vi "Save SCH FPGA Config Parameters to File MGI RWA.vi"(8 "error in (no error)":errorcluster, 11 "Refnum in":T2) -> (0 "error out":errorcluster, 2 "FPGA Configuration Values":T1={"Ln2 Filter Size"=10, "VT Quench Tick Limit"=4000000, "VT Quench Volt Limit"=0.1000061035156, "Joint Tick Limit"=4000000, "Joint Volt Limit"=0.0002000033855438, "CoWound Volt Limit"=0.2000122070312, "CoWound Tick Limit"=4000000, "SC Bus Limit"=0.0004000067710876, "SC Bus Tick Limit"=4000000, "ResMag Tick Limit"=1000000, "DAQ Cycle Ticks"=4096, "Res Mag dI/dt Delay"=256, "dI/dT scaling"=38.14697265625, "Pressure Inlet Limit (BarA)"=6.0, "Bore Tube Volt Limit"=0.5999999940395, "Pressure Outlet Limit (BarA)"=5.0, "Activation Current (kA)"=0.5, "Dump Resistor Scale Factor"=204.7939999998, "Co-Wound Asymmetry Factor"=-0.0026654, "Co-Wound Scale Factor"=60.04379999638, "Layer Scale Factors"=[4.000479996204, 3.501155003905, 3.50127799809, 3.501155003905, 3.001561000943, 3.001561000943, 3.50005300343, 3.500664994121, 3.501155003905, 4.000159993768, 3.999679997563, 4.000159993768, 3.998879998922, 3.999520003796, 3.999679997563, 4.000320002437, 4.00096000731, 4.000640004873], "Fudge Factors"=[0.0486624, 0.0491151, -0.0418637, -0.0149169, 0.0726134, -0.0451977, -0.0032112, -0.0234927, -0.002501, 0.0285479, -0.0270486, 0.003522, 0.0059306, -0.0088003, -0.0297659, 0.0390219], "Joint Scale Factors"=[0.0002005249261856, 0.0002005249261856, 0.0002004057168961, 0.000200480222702, 0.0002004057168961, 0.0002007633447647, 0.0002006888389587, 0.0002006441354752], "SC Bus Scale"=[0.09999999403954, 0.09999999403954, 0.001000002026558, 0.001000002026558, 0.0002005249261856, 0.0002006441354752], "Pressure Scale Factor"=[1.723690003157, 1.723690003157, 1.723690003157, 1.723690003157], "# Consecutive Zeros Fault"=1000, "Digitize Convert Ticks"=200, "Digitize Reset Ticks"=400, "Convert Clock Ticks"=20, "Digitize Read Delay Ticks"=38, "Digitize # Bits"=16, "HTS Lead Tick Limit"=4000000, "Res Lead Tick Limit"=4000000, "HTS Lead Trip"=0.1500000059605, "Res Lead Limit"=0.001953125, "HTS Lead FRZ"=0.006999999284744, "HTS Lead Warn"=0.001000002026558, "Low Current (kA)"=0.04500000178814, "Low Current Ticks"=400000000, "Low Current Delay Factor"=100, "HTS Resistance (nOhm)"=[0.0, 0.0], "Ticks to Close Relief"=80000000, "All Breaker Tick Limit"=400000000, "HTS Offset (microV)"=[0.0, 0.0], "Delay Ticks Between Bkr Reset"=1200000000, "Breaker Reset Ticks"=400000000, "PS Enable Reset Ticks"=400000000, "Reset Digitizer Ticks"=400000000, "Pressure Inlet Cooldown Limit"=12.0, "Pressure Outlet Cooldown Limit"=10.0, "Notification Email"="sth@magnet.fsu.edu"} {"Pressure Outlet Cooldown Limit" format="%.5g"; "Pressure Inlet Cooldown Limit" format="%.5g"; "HTS Offset (microV)" format="%_6g"; "HTS Resistance (nOhm)" format="%_6g"; "HTS Lead Warn" format="%_6g"; "HTS Lead FRZ" format="%_6g"; "Res Lead Limit" format="%_6g"; "HTS Lead Trip" format="%_6g"; "Pressure Scale Factor" format="%_6g"; "Joint Scale Factors" format="%_6g"; "Fudge Factors" format="%.7g"; "Co-Wound Asymmetry Factor" format="%.8g"; "Activation Current (kA)" format="%_6g"; "Pressure Outlet Limit (BarA)" format="%.5g"; "Bore Tube Volt Limit" format="%_6g"; "Pressure Inlet Limit (BarA)" format="%.5g"; "dI/dT scaling" format="%.11g"; "SC Bus Limit" format="%_6g"; "Joint Volt Limit" format="%_6g"; "VT Quench Volt Limit" format="%.5g"}, 3 "Refnum out":T2)   [LabVIEW 2021]
doc: "Author: Scott Hannahs <sth@magnet.fsu.edu>\nCopyright 2018 Florida State University, All rights reserved."
uses:
  RT Controls/FPGA SCH Digitizer Ref.ctl
  SCH Data Controls/FPGA Configure Parameters.ctl
  <userlib>/_MGI/Read Write Anything/MGI RWA Options Cluster.ctl
  <vilib>/Utility/error.llb/Error Cluster From Error Code.vi
  <vilib>/rvi/errors/niLvFpgaAdjustHostInterfaceError.vi
  RT Server Sub VIs/RT Host Globals.vi
  <vilib>/rvi/interface/nirviReadWriteControl/nirviReadWriteControl.xnode
  NiFpgaLv.dll
  <vilib>/rvi/interface/Simulation/niFpgaSimulationCallBeginRW.vi
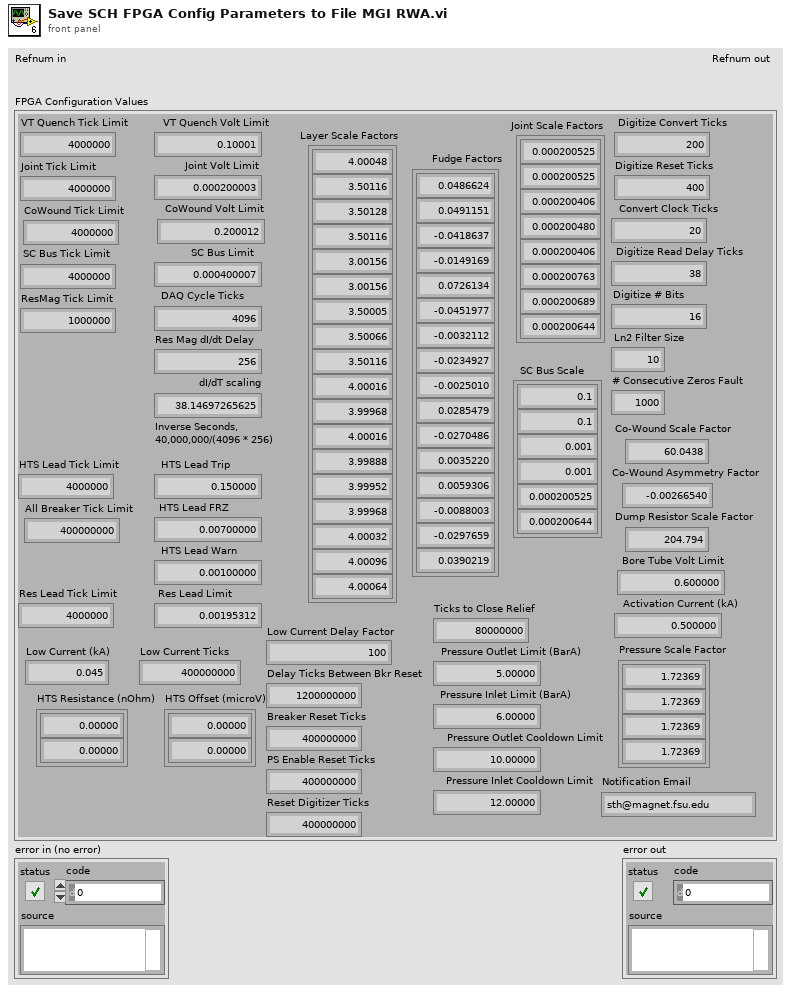
[diagram p1: front panel]
types:
  T1 = typedef "FPGA Configure Parameters.ctl" = cluster{"Ln2 Filter Size":i16, "VT Quench Tick Limit":u32, "VT Quench Volt Limit":dbl, "Joint Tick Limit":u32, "Joint Volt Limit":dbl, "CoWound Volt Limit":dbl, "CoWound Tick Limit":u32, "SC Bus Limit":dbl, "SC Bus Tick Limit":u32, "ResMag Tick Limit":u32, "DAQ Cycle Ticks":u32, "Res Mag dI/dt Delay":u32, "dI/dT scaling":dbl, "Pressure Inlet Limit (BarA)":dbl, "Bore Tube Volt Limit":dbl, "Pressure Outlet Limit (BarA)":dbl, "Activation Current (kA)":dbl, "Dump Resistor Scale Factor":dbl, "Co-Wound Asymmetry Factor":dbl, "Co-Wound Scale Factor":dbl, "Layer Scale Factors":dbl[], "Fudge Factors":dbl[], "Joint Scale Factors":dbl[], "SC Bus Scale":dbl[], "Pressure Scale Factor":dbl[], "# Consecutive Zeros Fault":i16, "Digitize Convert Ticks":u32, "Digitize Reset Ticks":u32, "Convert Clock Ticks":u32, "Digitize Read Delay Ticks":u32, "Digitize # Bits":u32, "HTS Lead Tick Limit":u32, "Res Lead Tick Limit":u32, "HTS Lead Trip":dbl, "Res Lead Limit":dbl, "HTS Lead FRZ":dbl, "HTS Lead Warn":dbl, "Low Current (kA)":dbl, "Low Current Ticks":u32, "Low Current Delay Factor":u16, "HTS Resistance (nOhm)":dbl[], "Ticks to Close Relief":u32, "All Breaker Tick Limit":u32, "HTS Offset (microV)":dbl[], "Delay Ticks Between Bkr Reset":u32, "Breaker Reset Ticks":u32, "PS Enable Reset Ticks":u32, "Reset Digitizer Ticks":u32, "Pressure Inlet Cooldown Limit":dbl, "Pressure Outlet Cooldown Limit":dbl, "Notification Email":string}
  T2 = typedef "FPGA SCH Digitizer Ref.ctl" = refnum<k20>
  T3 = typedef "MGI RWA Options Cluster.ctl" = cluster{"TS Fmt":string, "Int Fmt":string, "Delimiter":string}
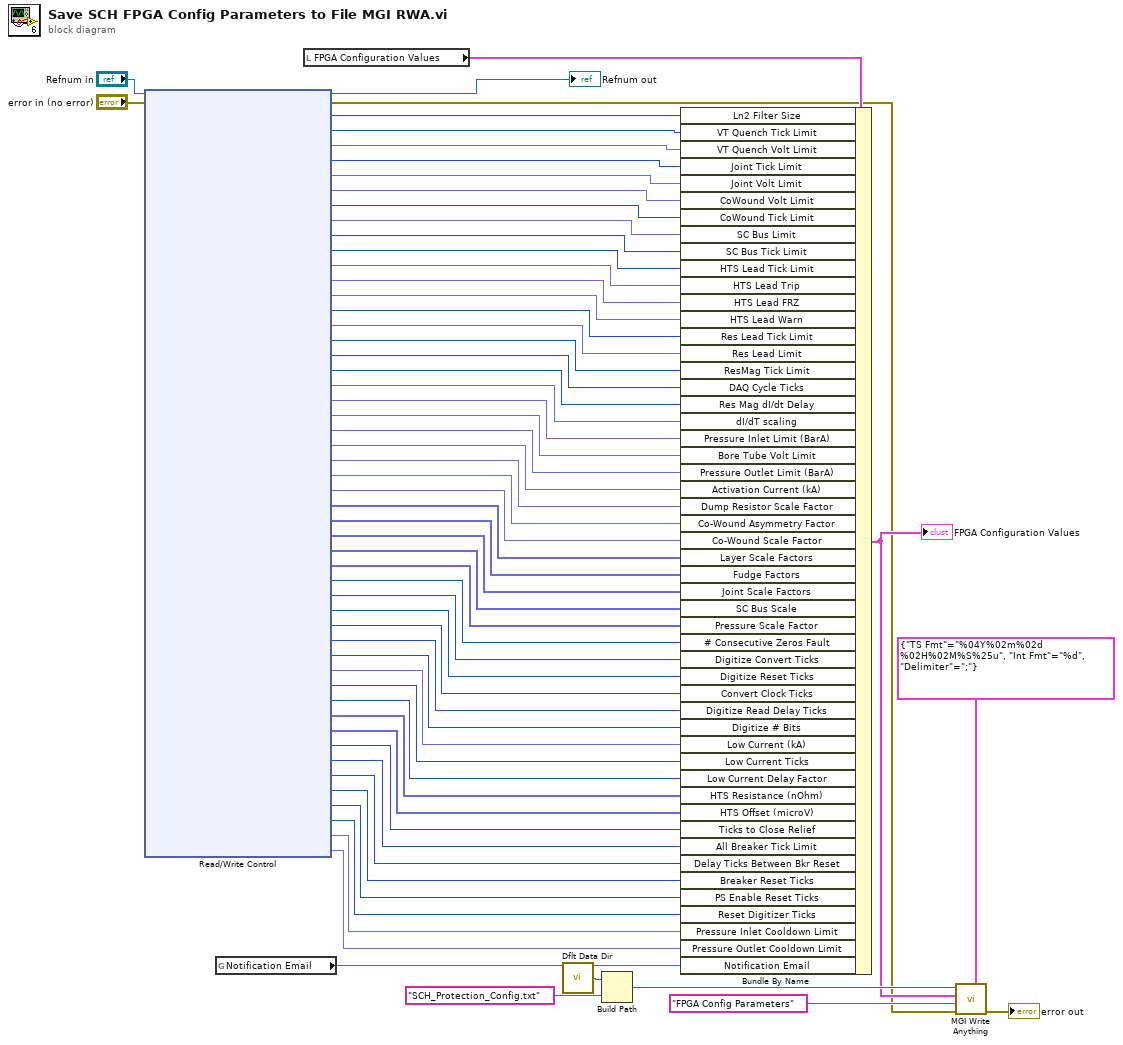
[diagram p0: block diagram]
diagram:
  n1 = xnode "Read/Write Control"("FPGA VI Reference In"="Refnum in", "error in"="error in (no error)") -> ("FPGA VI Reference Out"=→"Refnum out":T2, "error out"=w22:errorcluster, "Ln2 Filter Size"=w60:i16, "VT Quench Tick Limit"=w59:u32, "VT Quench Volt Limit"=w58:fxp<+/-,38,12>, "Joint Tick Limit"=w57:u32, "Joint Volt Limit"=w56:fxp<+/-,38,12>, "CoWound Volt Limit"=w55:fxp<+/-,16,1>, "CoWound Tick Limit"=w54:u32, "SC Bus Limit"=w53:fxp<+/-,38,12>, "SC Bus Tick Limit"=w52:u32, "HTS Lead Tick Limit"=w21:u32, "HTS Lead Trip"=w16:fxp<+/-,38,12>, "HTS Lead FRZ"=w17:fxp<+/-,38,12>, "HTS Lead Warn"=w18:fxp<+/-,38,12>, "Res Lead Tick Limit"=w19:u32, "Res Lead Limit"=w20:fxp<+/-,38,12>, "ResMag Tick Limit"=w51:u32, "DAQ Cycle Ticks"=w50:u32, "Res Mag dI/dt Delay"=w49:u32, "dI/dT scaling"=w48:fxp<+/-,35,11>, "Pressure Inlet Limit (BarA)"=w47:fxp<+/-,38,12>, "Bore Tube Volt Limit"=w46:fxp<+/-,38,12>, "Pressure Outlet Limit (BarA)"=w45:fxp<+/-,38,12>, "Activation Current (kA)"=w44:fxp<+/-,38,12>, "Dump Resistor Scale Factor"=w43:fxp<+/-,38,12>, "Co-Wound Asymmetry Factor"=w42:fxp<+/-,16,0>, "Co-Wound Scale Factor"=w41:fxp<+/-,38,12>, "Layer Scale Factors"=w40:fxp<+/-,38,12>[], "Fudge Factors"=w39:fxp<+/-,32,3>[], "Joint Scale Factors"=w38:fxp<+/-,38,12>[], "SC Bus Scale"=w37:fxp<+/-,38,12>[], "Pressure Scale Factor"=w36:fxp<+/-,38,12>[], "# Consecutive Zeros Fault"=w35:i16, "Digitize Convert Ticks"=w31:u32, "Digitize Reset Ticks"=w30:u32, "Convert Clock Ticks"=w29:u32, "Digitize Read Delay Ticks"=w28:u32, "Digitize # Bits"=w27:u32, "Low Current (kA)"=w14:fxp<+/-,38,12>, "Low Current Ticks"=w13:u32, "Low Current Delay Factor"=w12:u16, "HTS Resistance (nOhm)"=w11:fxp<+/-,38,12>[], "HTS Offset (microV)"=w9:fxp<+/-,38,12>[], "Ticks to Close Relief"=w10:u32, "All Breaker Tick Limit"=w8:u32, "Delay Ticks Between Bkr Reset"=w7:u32, "Breaker Reset Ticks"=w6:u32, "PS Enable Reset Ticks"=w5:u32, "Reset Digitizer Ticks"=w4:u32, "Pressure Inlet Cooldown Limit"=w3:fxp<+/-,38,12>, "Pressure Outlet Cooldown Limit"=w2:fxp<+/-,38,12>)
  n2 = global read "RT Host Globals.vi" "Notification Email"() -> (w1:string)
  n3 = local read "FPGA Configuration Values"() -> (w34:T1)
  n4 = call <vilib>:"Dflt Data Dir.vi"() -> ("App:Default Data Directory"=w32:path)
  n5 = Build Path(base path=w32, name or relative path="SCH_Protection_Config.txt") -> (appended path=w26:path)
  n6 = Bundle By Name(cluster=w34, "Ln2 Filter Size"=w60, "VT Quench Tick Limit"=w59, "VT Quench Volt Limit"=w58, "Joint Tick Limit"=w57, "Joint Volt Limit"=w56, "CoWound Volt Limit"=w55, "CoWound Tick Limit"=w54, "SC Bus Limit"=w53, "SC Bus Tick Limit"=w52, "HTS Lead Tick Limit"=w21, "HTS Lead Trip"=w16, "HTS Lead FRZ"=w17, "HTS Lead Warn"=w18, "Res Lead Tick Limit"=w19, "Res Lead Limit"=w20, "ResMag Tick Limit"=w51, "DAQ Cycle Ticks"=w50, "Res Mag dI/dt Delay"=w49, "dI/dT scaling"=w48, "Pressure Inlet Limit (BarA)"=w47, "Bore Tube Volt Limit"=w46, "Pressure Outlet Limit (BarA)"=w45, "Activation Current (kA)"=w44, "Dump Resistor Scale Factor"=w43, "Co-Wound Asymmetry Factor"=w42, "Co-Wound Scale Factor"=w41, "Layer Scale Factors"=w40, "Fudge Factors"=w39, "Joint Scale Factors"=w38, "SC Bus Scale"=w37, "Pressure Scale Factor"=w36, "# Consecutive Zeros Fault"=w35, "Digitize Convert Ticks"=w31, "Digitize Reset Ticks"=w30, "Convert Clock Ticks"=w29, "Digitize Read Delay Ticks"=w28, "Digitize # Bits"=w27, "Low Current (kA)"=w14, "Low Current Ticks"=w13, "Low Current Delay Factor"=w12, "HTS Resistance (nOhm)"=w11, "HTS Offset (microV)"=w9, "Ticks to Close Relief"=w10, "All Breaker Tick Limit"=w8, "Delay Ticks Between Bkr Reset"=w7, "Breaker Reset Ticks"=w6, "PS Enable Reset Ticks"=w5, "Reset Digitizer Ticks"=w4, "Pressure Inlet Cooldown Limit"=w3, "Pressure Outlet Cooldown Limit"=w2, "Notification Email"=w1) -> (w24:T1)
  "FPGA Configuration Values" <- w24
  n7 = call <userlib>:"MGI Write Anything.vi"("Read/Write Options"=T3 {"TS Fmt"="%04Y%02m%02d %02H%02M%S%25u", "Int Fmt"="%d", "Delimiter"=";"}, "Error In"=w22, "Section Name (Name of \"Anything\")"="FPGA Config Parameters" ("section"), "Anything"=w24, "Path (dialog)"=w26) -> ("Error Out"=→"error out":errorcluster)  [unwired: 4 in, 2 out]
